vi "Read Data.vi"(0 "Caraya Unit Test in":refnum<class "Caraya Test.lvclass">, 11 "error in (no error)":errorcluster) -> (2 "Report Extension":string, 3 "Report Name Override":string, 4 "Caraya Unit Test out":refnum<class "Caraya Test.lvclass">, 6 "Target Name":string, 8 "Verbose":bool, 10 "Relative Project Override Path":string, 14 "Timeout":i32, 15 "error out":errorcluster)   [LabVIEW 2019, in "ProjectBuilder.lvlib" / "Caraya Test.lvclass"]
doc: "Read private data."
uses:
  Caraya Test.lvclass
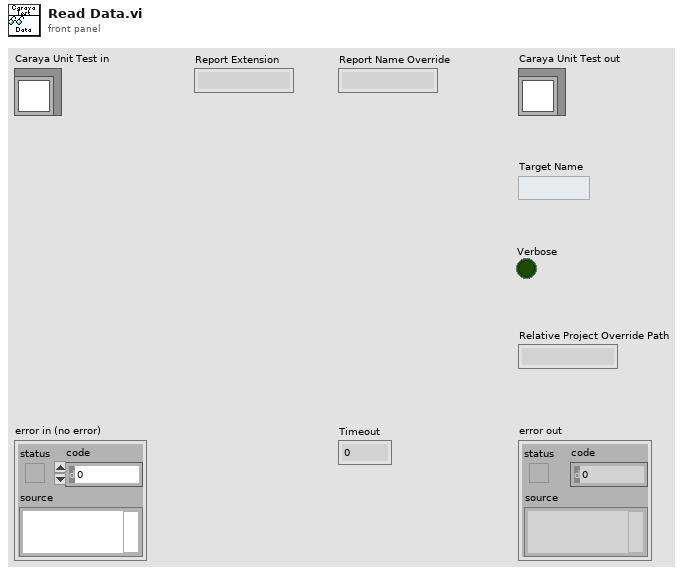
[diagram p1: front panel]
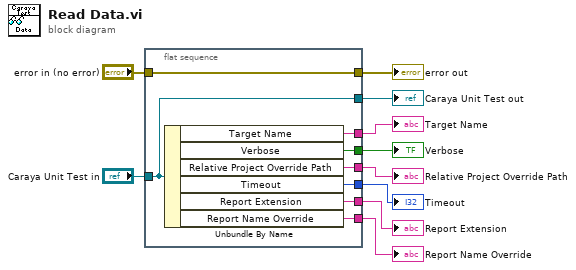
[diagram p0: block diagram]
diagram:
  n1 = flat-sequence {
    tunnel: "error in (no error)" -> [w18]
    tunnel: [w18] -> w9
    tunnel: "Caraya Unit Test in" -> [w17]
    tunnel: [w17] -> w7
    tunnel: [w16] -> w6
    tunnel: [w15] -> w5
    tunnel: [w14] -> w4
    tunnel: [w13] -> w3
    tunnel: [w12] -> w2
    tunnel: [w11] -> w1
    frame #0 {
      n2 = Unbundle By Name(w17) -> ("Target Name"=w16:string, "Verbose"=w11:bool, "Relative Project Override Path"=w12:string, "Timeout"=w13:i32, "Report Extension"=w14:string, "Report Name Override"=w15:string)
    }
  }
  "error out" <- w9
  "Caraya Unit Test out" <- w7
  "Target Name" <- w6
  "Verbose" <- w1
  "Relative Project Override Path" <- w2
  "Timeout" <- w3
  "Report Extension" <- w4
  "Report Name Override" <- w5
